vi "Write To Spreadsheet File with err check.vi"(4 "transpose? (no:F)":bool, 5 "format (%.3f)":string="%.3f", 6 "error in (no error)":errorcluster, 7 "delimiter (Tab)":string="\t", 8 "append to file? (new file:F)":bool, 9 "1D data":dbl[](array[numeric]) format="%.2f", 10 "2D data":dbl[][](array[numeric]) format="%.2f", 11 "file path (dialog if empty)":path) -> (0 "error out":errorcluster, 3 "new file path (Not A Path if cancelled)":path)   [LabVIEW 2015]
doc: "Converts a 2D or 1D array of single-precision numbers to a text string and writes the string to a new byte stream file or appends the string to an existing file."
panel:
  in  "prompt":string="Choose file to write."
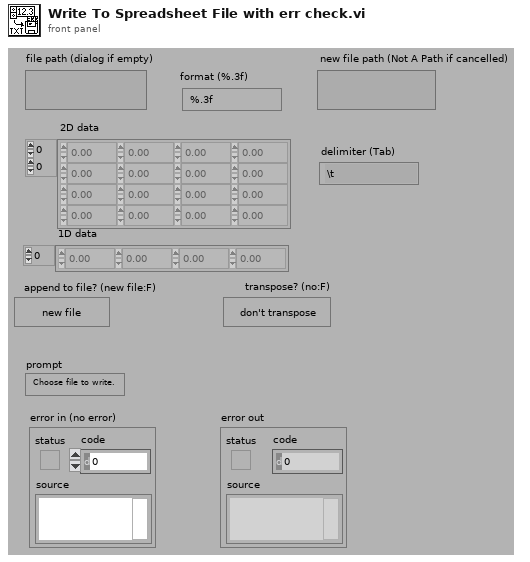
[diagram p1: front panel]
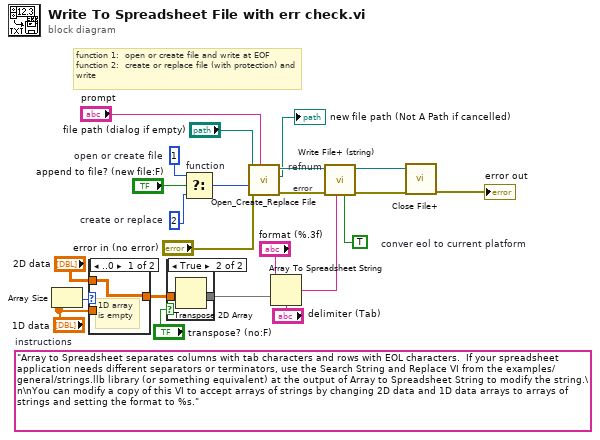
[diagram p0: block diagram]
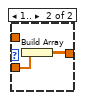
[diagram p3: hidden frame]
diagram:
  (unwired) "Array to Spreadsheet separates columns with tab characters and rows with EOL characters.  If your spreadsheet application needs different separators or terminators, use the Search String and Replace VI from the examples/general/strings.llb library (or something equivalent) at the output of Array to Spreadsheet String to modify the string.\n\nYou can modify a copy of this VI to accept arrays of strings by changing 2D data and 1D data arrays to arrays of strings and setting the format to %s."  # instructions
  w5 = i16 2  # create or replace
  w8 = TRUE  # conver eol to current platform
  w22 = i16 1  # open or create file
  # "error"
  # "refnum"
  # "function 1:  open or create file and write at EOF\nfunction 2:  create or replace file (with protection) and write"
  n1 = Array Size(array="1D data") -> (size(s)=w20:i32)
  n2 = case shown="..0" w20 {
    tunnel: "1D data" -> [_ w26]
    tunnel: [w24 w25] -> w16
    tunnel: "2D data" -> [w24 _]
    frame ..0 {
      # "1D array is empty"
    }
    frame 1.. {
      n3 = Build Array(w26) -> (w25:dbl[][])
    }
  }
  n4 = case shown="True" "transpose? (no:F)" {
    tunnel: [w27 w29] -> w14
    tunnel: w16 -> [w27 w28]
    frame False {
    }
    frame True {
      n5 = Transpose 2D Array(2D array=w28) -> (transposed array=w29:dbl[][])
    }
  }
  n6 = Select "function"(t=w22, s="append to file? (new file:F)", f=w5) -> (s? t:f=w13:i16)
  n7 = call <vilib>:"Open_Create_Replace File.vi"("prompt"="prompt", "error in (no error)"="error in (no error)", "function (open:0)"=w13, "file path"="file path (dialog if empty)") -> ("error out"=w11:errorcluster, "new file path"=→"new file path (Not A Path if cancelled)":path, "refnum"=w7:refnum<file>)  [unwired: 2 in, 3 out]
  n8 = Array To Spreadsheet String(delimiter (Tab)="delimiter (Tab)", array=w14, 3:"format (%.3f)") -> (spreadsheet string=w10:string)
  n9 = call <vilib>:"Write File+ (string).vi"("convert eol? (no:F)"=w8, "string"=w10, "error in (no error)"=w11, "refnum"=w7) -> ("error out"=w21:errorcluster, "dup refnum"=w9:refnum<file>)  [unwired: 2 in, 2 out]
  n10 = call <vilib>:"Close File+.vi"("error in (no error)"=w21, "refnum"=w9) -> ("error out"=→"error out":errorcluster)  [unwired: 5 out]
